vi "BioFeedback(DAQ+FlowControl).vi"() -> ()   [LabVIEW 2016]
uses:
  <vilib>/Analysis/5stat.llb/RMS (DBL).vi
  <vilib>/Waveform/WDTOps.llb/WDT Append Waveforms DBL.vi
  <vilib>/Waveform/WDTFileIO.llb/ Write Waveform to File.vi
  <vilib>/Analysis/NI_AALPro.lvlib
panel:
  in  "VR Percent Path":path
  in  "Target Percentage":dbl
  in  "Base Directory":path
  out "Trial Data":waveform(dbl)
  out "Trial In Progress":bool
  in  "End Trial":bool
  in  "Start Trial":bool
  in  "Trial Number":dbl
  in  "MARK":bool
  in  "Save Data":bool
  in  "File Postfix":string
  in  "Folder Name":string
  in  "VR Data Input File":path
  out "Moving Avg\n RMS Graph":dbl(graph)
  out "Moving Avg RMS":dbl(slide) scale=0.0..0.07
  out "Rectified Moving\nAverage Sample":waveform(dbl)[](graph)
  out "Filtered data":waveform(dbl)
  in  "Lower Cut-Off":dbl=20.0
  in  "Upper Cut-Off":dbl=300.0
  out "raw data":dynamicdata(graph)
  out "Bufffer Index":dbl
  out "Frames in Buffer":dbl
  out "Samples per frame":dbl
  out "AggregateSignalData":waveform(dbl)[](array[waveform])
  out "Reset Data Acquisition\nAnd UI Updating":bool=TRUE
  in  "Moving Average Length (s)":dbl
  in  "Frames Per Second":dbl
  in  "Sample rate (Hz)":dbl=22050.0
  in  "End Program":bool
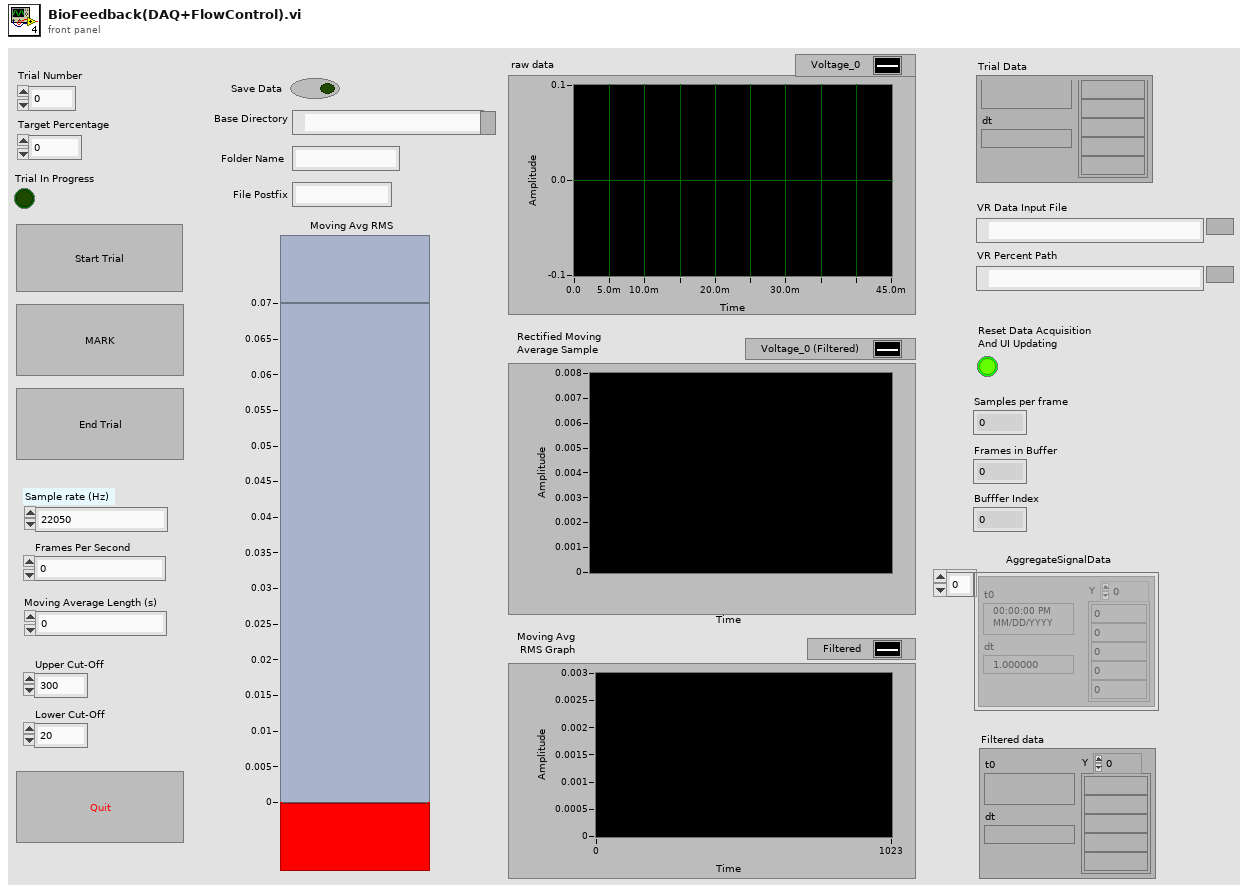
[diagram p1: front panel]
types:
  T1 = typedef "WaveformArrayControl.ctl" = waveform(dbl)[]
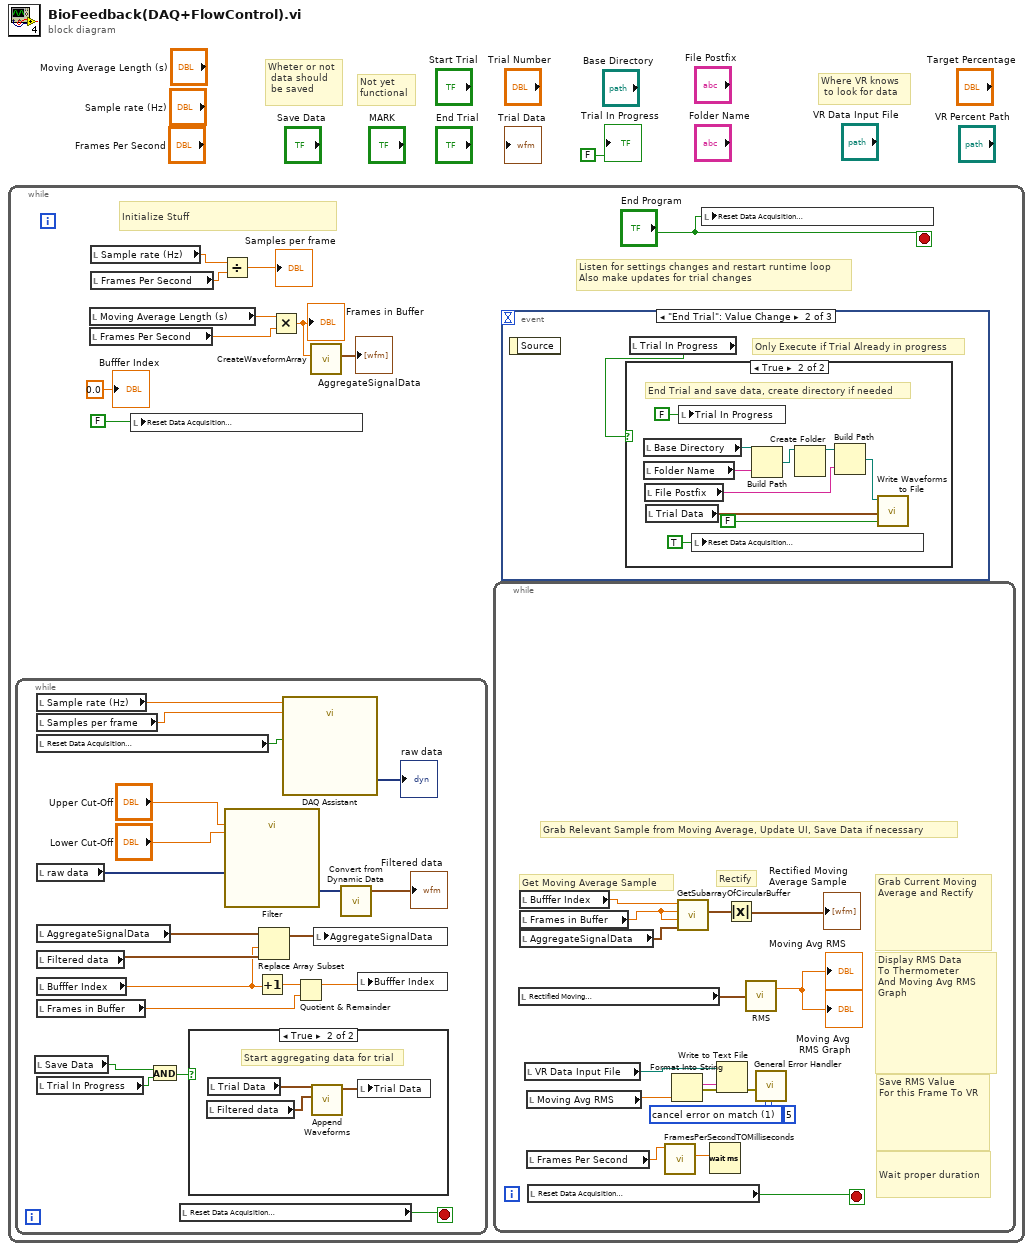
[diagram p0: block diagram]
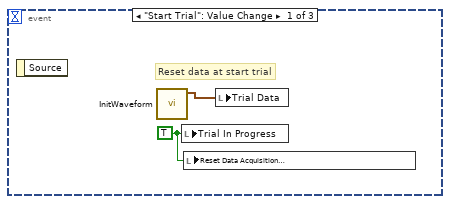
[diagram p2: hidden frame]
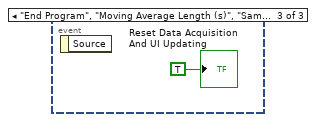
[diagram p4: hidden frame]
diagram:
  # "Not yet \nfunctional"
  # "Wheter or not\n data should\n be saved"
  # "Where VR knows\n to look for data"
  n1 = while {
    stop <- "End Program" stop-if-true
    # "Grab Relevant Sample from Moving Average, Update UI, Save Data if necessary"
    # "Initialize Stuff"
    # "Listen for settings changes and restart runtime loop\nAlso make updates for trial changes"
    n2 = while {
      stop <- w47 stop-if-true
      n3 = local read "Save Data"() -> (w44:bool)
      n4 = local read "Sample rate (Hz)"() -> (w62:dbl)
      n5 = local read "Samples per frame"() -> (w61:dbl)
      n6 = local read "Reset Data Acquisition\nAnd UI Updating"() -> (w46:bool)
      n7 = local read "raw data"() -> (w59:dynamicdata)
      n8 = local read "AggregateSignalData"() -> (w54:waveform(dbl)[])
      n9 = local read "Filtered data"() -> (w53:waveform(dbl))
      n10 = local read "Bufffer Index"() -> (w52:dbl)
      n11 = local read "Frames in Buffer"() -> (w49:dbl)
      n12 = local read "Trial In Progress"() -> (w45:bool)
      n13 = And(x=w44, y=w45) -> (x .and. y?=w43:bool)
      n14 = local read "Reset Data Acquisition\nAnd UI Updating"() -> (w47:bool)
      n15 = case shown="True" w43 {
        frame False {
        }
        frame True {
          # "Start aggregating data for trial"
          n16 = local read "Filtered data"() -> (w64:waveform(dbl))
          n17 = local read "Trial Data"() -> (w65:waveform(dbl))
          n18 = call-poly <vilib>:"Append Waveforms.vi"("waveform B"=w64, "waveform A"=w65) -> ("waveform out"=w63:waveform(dbl))  [unwired: 8 in, 1 out]
          n19 = local write "Trial Data"(w63) -> ()
        }
      }
      n20 = call "Filter"("Lower Cut-Off"="Lower Cut-Off", "Upper Cut-Off"="Upper Cut-Off", "Signal"=w59) -> ("Filtered Signal"=w56:dynamicdata)  [unwired: 7 in, 1 out]
      n21 = Increment(x=w52) -> (x+1=w48:dbl)
      n22 = Replace Array Subset(array=w54, new element=w53, index=w52) -> (w51:waveform(dbl)[])
      n23 = call "DAQ Assistant"("rate"=w62, "number of samples"=w61, "stop (T)"=w46) -> ("data"=→"raw data":dynamicdata)  [unwired: 14 in, 2 out]
      n24 = Quotient & Remainder(x=w48, y=w49) -> (x-y*floor(x/y)=w50:dbl)  [unwired: 1 out]
      n25 = local write "AggregateSignalData"(w51) -> ()
      n26 = call "Convert from Dynamic Data"("Dynamic Data Type"=w56) -> ("Waveform"=→"Filtered data":waveform(dbl))  [unwired: 3 in]
      n27 = local write "Bufffer Index"(w50) -> ()
    }
    n28 = local read "Moving Average Length (s)"() -> (w8:dbl)
    n29 = local read "Frames Per Second"() -> (w7:dbl)
    n30 = local read "Sample rate (Hz)"() -> (w11:dbl)
    n31 = local read "Frames Per Second"() -> (w10:dbl)
    n32 = local write "Reset Data Acquisition\nAnd UI Updating"(FALSE) -> ()
    n33 = Divide(x=w11, y=w10) -> (x/y=→"Samples per frame":dbl)
    n34 = Multiply(x=w8, y=w7) -> (x*y=w2:dbl)
    "Frames in Buffer" <- w2
    n35 = call "CreateWaveformArray.vi"("bufferSize"=w2) -> ("initialized array"=→"AggregateSignalData":waveform(dbl)[])  [unwired: 5 in, 1 out]
    n36 = while {
      stop <- w42 stop-if-true
      w32 = 1 items=["no exception", "cancel error on match", "set error on match"] ("[exception action] (none:0)")
      # "Wait proper duration"
      # "Save RMS Value\nFor this Frame To VR"
      # "Display RMS Data\nTo Thermometer\nAnd Moving Avg RMS\nGraph"
      # "Grab Current Moving\nAverage and Rectify"
      # "Get Moving Average Sample"
      # "Rectify"
      n37 = local read "Rectified Moving\nAverage Sample"() -> (w35:waveform(dbl)[])
      n38 = local read "Bufffer Index"() -> (w41:dbl)
      n39 = local read "Frames in Buffer"() -> (w40:dbl)
      n40 = local read "AggregateSignalData"() -> (w39:waveform(dbl)[])
      n41 = local read "VR Data Input File"() -> (w28:path)
      n42 = local read "Moving Avg RMS"() -> (w26:dbl)
      n43 = local read "Frames Per Second"() -> (w34:dbl)
      n44 = local read "Reset Data Acquisition\nAnd UI Updating"() -> (w42:bool)
      n45 = call "FramesPerSecondTOMilliseconds.vi"("Thermometer\nFps"=w34) -> ("x*y"=w33:dbl)  [unwired: 10 in]
      n46 = Format Into String(w26) -> (resulting string=w27:string, error out=w29:errorcluster)  [unwired: 3 in]
      n47 = call "GetSubarrayOfCircularBuffer.vi"("initialized array"=w39, "buffer size"=w40, "subset size"=w40, "start index"=w41) -> ("initialized array 2"=w38:T1)  [unwired: 7 in]
      n48 = Wait (ms)(milliseconds to wait=w33) -> ()  [unwired: 1 out]
      n49 = Write to Text File(file (use dialog)=w28, text=w27, error in=w29) -> (error out=w30:errorcluster)  [unwired: 1 in, 2 out]
      n50 = Absolute Value(x=w38) -> (abs(x)=→"Rectified Moving\nAverage Sample":T1)
      n51 = call-poly <vilib>:"RMS.vi"("X"=w35) -> ("rms value"=→"Moving Avg RMS" →"Moving Avg\n RMS Graph":dbl)  [unwired: 1 out]
      n52 = call <vilib>:"General Error Handler.vi"("error in (no error)"=w30, "[exception action] (none:0)"=w32, "[exception code]"=5) -> ()  [unwired: 8 in, 5 out]
    }
    n53 = event shown="[1] \"End Trial\": Value Change" {
      selector: _ -> [_ _ _]
      dyn-events: _ -> [_ _ _]
      timeout: _ -> [_ _ _]
      event "Start Trial": Value Change {
        w12 = TRUE ("Trial In Progress")
        # "Reset data at start trial"
        n54 = event-data() -> ()  [unwired: 1 in, 1 out]
        n55 = call "InitWaveform.vi"() -> ("output waveform"=w13:waveform(dbl))  [unwired: 11 in]
        n56 = local write "Trial In Progress"(w12) -> ()
        n57 = local write "Reset Data Acquisition\nAnd UI Updating"(w12) -> ()
        n58 = local write "Trial Data"(w13) -> ()
      }
      event "End Trial": Value Change {
        # "Only Execute if Trial Already in progress"
        n59 = event-data() -> ()  [unwired: 1 in, 1 out]
        n60 = local read "Trial In Progress"() -> (w14:bool)
        n61 = case shown="True" w14 {
          frame False {
          }
          frame True {
            # "End Trial and save data, create directory if needed"
            n62 = local read "Base Directory"() -> (w19:path)
            n63 = local read "Folder Name"() -> (w20:string)
            n64 = local read "File Postfix"() -> (w23:string)
            n65 = local read "Trial Data"() -> (w17:waveform(dbl))
            n66 = local write "Trial In Progress"(FALSE ("Trial In Progress")) -> ()
            n67 = local write "Reset Data Acquisition\nAnd UI Updating"(TRUE ("Reset Data Acquisition\nAnd UI Updating")) -> ()
            n68 = Build Path(base path=w19, name or relative path=w20) -> (appended path=w21:path)
            n69 = Create Folder(path (use dialog)=w21) -> (created path=w22:path)  [unwired: 2 in, 2 out]
            n70 = Build Path(base path=w22, name or relative path=w23) -> (appended path=w24:path)
            n71 = call-poly <vilib>:"Write Waveforms to File.vi"("append to file? (new file:F)"=FALSE, "waveform"=w17, "file path (dialog if empty)"=w24) -> ()  [unwired: 7 in, 2 out]
          }
        }
      }
      event "End Program", "Moving Average Length (s)", "Sample rate (Hz)", "Frames Per Second": Value Change {
        n72 = event-data() -> ()  [unwired: 1 in, 1 out]
        "Reset Data Acquisition\nAnd UI Updating" <- TRUE
      }
    }
    n73 = local write "Reset Data Acquisition\nAnd UI Updating"("End Program") -> ()
    "Bufffer Index" <- 0.0 ("Bufffer Index")
  }
  "Trial In Progress" <- FALSE ("Trial In Progress")
